vi "IB_RW_Project_RegDest.vi"(7 "action":T3, 8 "error in (no error)":errorcluster, 9 "index in":string, 10 "RegDest":T2, 11 "buildObject":T1) -> (0 "error out":errorcluster, 1 "index out":string, 2 "RegDest":T2, 3 "buildObject out":T1)   [LabVIEW 2020]
doc: "Reads and writes the data to the object property bag."
uses:
  <resource>/Framework/Providers/API/ItemRef.ctl
  <vilib>/AppBuilder/IB_RW_Project/IB_RW_Project_RegDest_Data.ctl
  <vilib>/AppBuilder/IB_RW_Project/IB_RW_Project_PropBag_Action.ctl
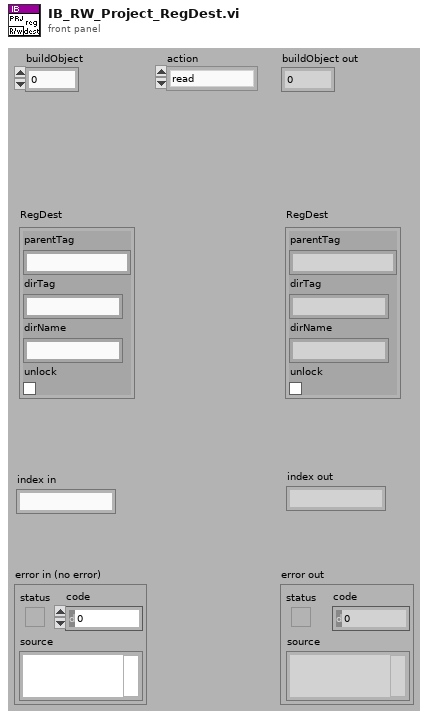
[diagram p1: front panel]
types:
  T1 = typedef "ItemRef.ctl" = u64
  T2 = typedef "IB_RW_Project_RegDest_Data.ctl" = cluster{"parentTag":string, "dirTag":string, "dirName":string, "unlock":bool}
  T3 = typedef "IB_RW_Project_PropBag_Action.ctl" = enum16{"read", "write", "clear", "readPrevious", "writePrevious", "clearPrevious"}
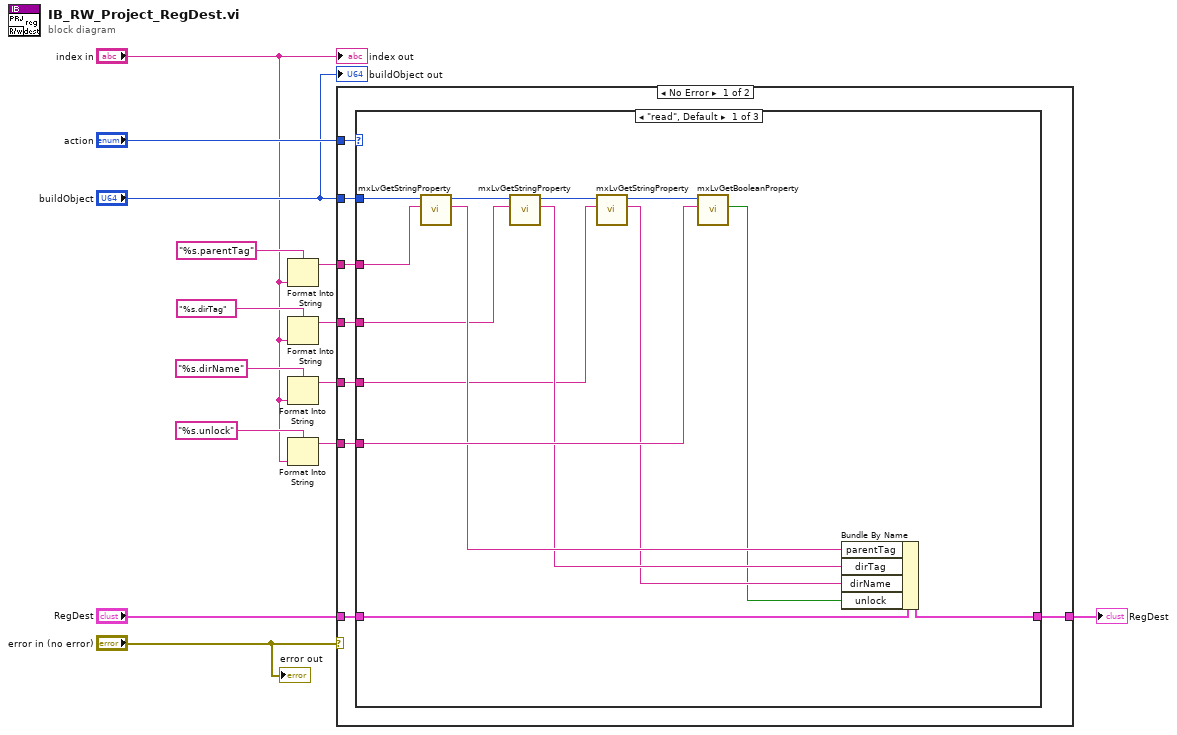
[diagram p0: block diagram]
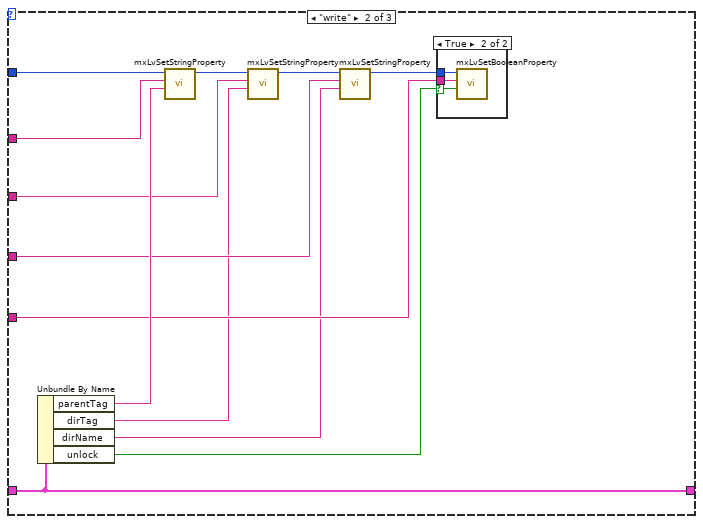
[diagram p2: hidden frame]
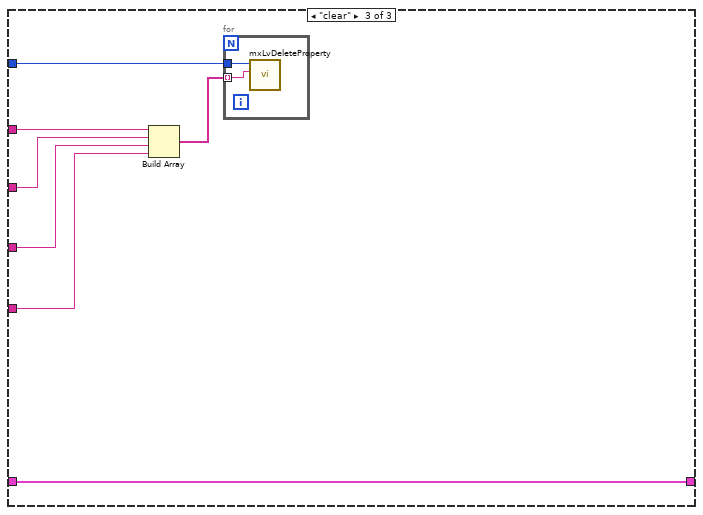
[diagram p4: hidden frame]
diagram:
  n1 = Format Into String(format string="%s.parentTag", "index in") -> (resulting string=w11:string)  [unwired: 2 in, 1 out]
  n2 = Format Into String(format string="%s.dirTag", "index in") -> (resulting string=w4:string)  [unwired: 2 in, 1 out]
  n3 = Format Into String(format string="%s.dirName", "index in") -> (resulting string=w2:string)  [unwired: 2 in, 1 out]
  n4 = Format Into String(format string="%s.unlock", "index in") -> (resulting string=w6:string)  [unwired: 2 in, 1 out]
  n5 = case shown="No Error" "error in (no error)" {
    tunnel: "action" -> [w22 _]
    tunnel: "RegDest" -> [w21 w62]
    tunnel: w11 -> [w20 _]
    tunnel: [w19 w62] -> w10
    tunnel: "buildObject" -> [w18 _]
    tunnel: w6 -> [w17 _]
    tunnel: w4 -> [w16 _]
    tunnel: w2 -> [w15 _]
    frame No Error {
      n6 = case shown="\"read\", Default" w22 {
        tunnel: w18 -> [w34 w48 w53]
        tunnel: w21 -> [w36 w49 w59]
        tunnel: w20 -> [w33 w47 w58]
        tunnel: [w35 w49 w59] -> w19
        tunnel: w17 -> [w32 w45 w54]
        tunnel: w16 -> [w29 w40 w56]
        tunnel: w15 -> [w26 w39 w55]
        frame "read", Default {
          n7 = call <resource>:"mxLvGetStringProperty.vi"("Tag"=w33, "Item"=w34) -> ("Value"=w31:string, "Item"=w30:T1)  [unwired: 1 in, 7 out]
          n8 = call <resource>:"mxLvGetStringProperty.vi"("Tag"=w29, "Item"=w30) -> ("Value"=w28:string, "Item"=w27:T1)  [unwired: 1 in, 7 out]
          n9 = call <resource>:"mxLvGetStringProperty.vi"("Tag"=w26, "Item"=w27) -> ("Value"=w25:string, "Item"=w24:T1)  [unwired: 1 in, 7 out]
          n10 = call <resource>:"mxLvGetBooleanProperty.vi"("Tag"=w32, "Item"=w24) -> ("Value"=w23:bool)  [unwired: 1 in, 8 out]
          n11 = Bundle By Name(cluster=w36, "parentTag"=w31, "dirTag"=w28, "dirName"=w25, "unlock"=w23) -> (w35:T2)
        }
        frame "write" {
          n12 = Unbundle By Name(w49) -> ("parentTag"=w46:string, "dirTag"=w38:string, "dirName"=w37:string, "unlock"=w44:bool)
          n13 = call <resource>:"mxLvSetStringProperty.vi"("Value (\"\")"=w46, "Tag"=w47, "Item"=w48) -> ("Item"=w43:T1)  [unwired: 2 in, 6 out]
          n14 = call <resource>:"mxLvSetStringProperty.vi"("Value (\"\")"=w38, "Tag"=w40, "Item"=w43) -> ("Item"=w42:T1)  [unwired: 2 in, 6 out]
          n15 = call <resource>:"mxLvSetStringProperty.vi"("Value (\"\")"=w37, "Tag"=w39, "Item"=w42) -> ("Item"=w41:T1)  [unwired: 2 in, 6 out]
          n16 = case shown="True" w44 {
            selector: w44 -> [_ w50]
            tunnel: w41 -> [_ w52]
            tunnel: w45 -> [_ w51]
            frame False {
            }
            frame True {
              n17 = call <resource>:"mxLvSetBooleanProperty.vi"("Value (F)"=w50, "Tag"=w51, "Item"=w52) -> ()  [unwired: 2 in, 7 out]
            }
          }
        }
        frame "clear" {
          n18 = Build Array(w58, w56, w55, w54) -> (w57:string[])
          n19 = for {
            tunnel: w57 -> [w61] mode=indexing
            tunnel: w53 -> [w60]
            n20 = call <resource>:"mxLvDeleteProperty.vi"("Tag"=w61, "Item"=w60) -> ()  [unwired: 1 in, 9 out]
          }
        }
      }
    }
    frame Error {
    }
  }
  "RegDest" <- w10
  "error out" <- "error in (no error)"
  "buildObject out" <- "buildObject"
  "index out" <- "index in"
